vi "locate channel refs.vi"(5 "Access":T2, 7 "Channel Type":T3, 8 "error in":errorcluster, 10 "Variant":variant, 11 "Device Reference in":T4 format="%.0x") -> (0 "error out":errorcluster, 3 "refs":T1[](array[typedef]) format="%.0x")   [LabVIEW 2015, in "Scriptable Model Interface Engine.lvlib"]
uses:
  Scriptable Model Interface Engine.lvlib
  <vilib>/NI Veristand/Custom Device API/Custom Device Item Ref.ctl
  <vilib>/NI Veristand/Custom Device API/Custom Device Channel Type.ctl
  <vilib>/NI Veristand/Custom Device API/Data Access Type.ctl
  <vilib>/NI Veristand/Custom Device API/Data Reference.ctl
  Shared/Scriptable Model Interface Shared.lvlib
  <vilib>/NI Veristand/Custom Device API/Custom Device API.lvlib
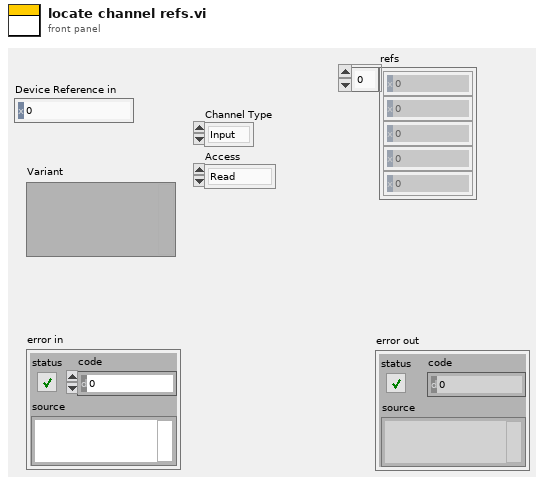
[diagram p1: front panel]
types:
  T1 = typedef "Custom Device API.lvlib/Data Reference.ctl" = i32
  T2 = typedef "Custom Device API.lvlib/Data Access Type.ctl" = enum16{"Read", "Write"}
  T3 = typedef "Custom Device API.lvlib/Custom Device Channel Type.ctl" = enum16{"Input", "Output"}
  T4 = typedef "Custom Device API.lvlib/Custom Device Item Ref.ctl" = u64
  T5 = typedef "Scriptable Model Interface Shared.lvlib/channel id.ctl" = cluster{"Name":string, "index":i32}
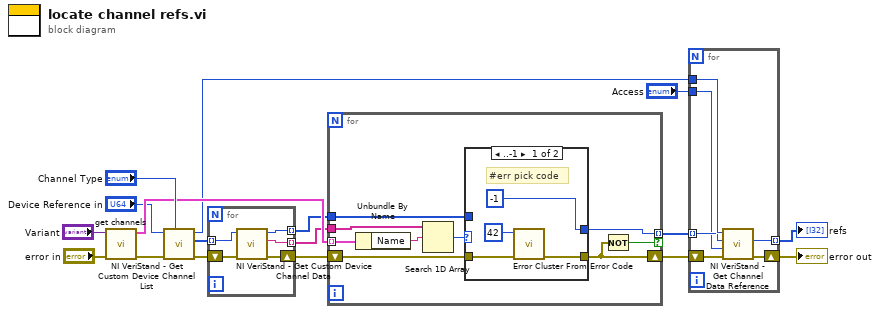
[diagram p0: block diagram]
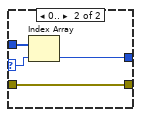
[diagram p2: hidden frame]
diagram:
  n1 = call "get channels.vi"("error in"="error in", "cluster in"="Variant") -> ("error out"=w15:errorcluster, "channels"=w10:T5[])  [unwired: 8 in]
  n2 = call <vilib>:"NI VeriStand - Get Custom Device Channel List.vi"("Channel Type"="Channel Type", "error in (no error)"=w15, "Device Ref in"="Device Reference in") -> ("error out"=w13:errorcluster, "Specified Channel Ref List"=w12:T4[], "Device Ref out"=w4:T4)  [unwired: 6 in]
  n3 = for {
    shift-right: [w20] -> w11
    shift-left: w13 -> [w22]
    tunnel: w12 -> [w21] mode=indexing
    tunnel: [w19] -> w9 mode=indexing
    tunnel: [w18] -> w8 mode=indexing
    n4 = call <vilib>:"NI VeriStand - Get Custom Device Channel Data.vi"("error in (no error)"=w22, "Channel Ref in"=w21) -> ("error out"=w20:errorcluster, "Channel Name"=w18:string, "Channel Ref out"=w19:T4)  [unwired: 4 in, 3 out]
  }
  n5 = for {
    shift-right: [w23] -> w6
    shift-left: w11 -> [w27]
    tunnel: w10 -> [w31] mode=indexing
    tunnel: w9 -> [w26]
    tunnel: w8 -> [w30]
    tunnel: [w25] -> w3 mode=indexing if=w24
    n6 = Unbundle By Name(w31) -> ("Name"=w29:string)
    n7 = Search 1D Array(1D array=w30, element=w29) -> (index of element=w28:i32)  [unwired: 1 in]
    n8 = case shown="..-1" w28 {
      selector: w28 -> [_ w38]
      tunnel: [w33 w36] -> w23
      tunnel: w27 -> [w35 w36]
      tunnel: w26 -> [_ w39]
      tunnel: [T1 -1 ("Channel Data Reference") w37] -> w25
      frame ..-1 {
        # "#err pick code"
        n9 = call <vilib>:"Error Cluster From Error Code.vi"("error in (no error)"=w35, "error code (0)"=42) -> ("error out"=w33:errorcluster)  [unwired: 7 in]
      }
      frame 0.. {
        n10 = Index Array(array=w39, index=w38) -> (element=w37:T4)
      }
    }
    n11 = Not(x=w23) -> (.not. x?=w24:bool)
  }
  n12 = for {
    tunnel: w4 -> [w43]
    tunnel: w3 -> [w42] mode=indexing
    tunnel: "Access" -> [w41]
    shift-right: [w44] -> w5
    shift-left: w6 -> [w45]
    tunnel: [w40] -> w1 mode=indexing
    n13 = call <vilib>:"NI VeriStand - Get Channel Data Reference.vi"("error in (no error)"=w45, "Access"=w41, "Channel Ref in"=w42, "Device Ref in"=w43) -> ("error out"=w44:errorcluster, "Channel Data Reference"=w40:T1)  [unwired: 5 in, 1 out]
  }
  "error out" <- w5
  "refs" <- w1
